vi "Custom Aggregation (Flags).vi"(0 "voltage flags? (F)":bool[](array[boolean]), 1 "reset? (F)":bool, 5 "aggregation settings":T1={"interval"=1, "interval unit"=enum."Runs", "synchronization of intervals"=enum."Not synchronized", "algorithm"=enum."Average"}, 9 "system info in":refnum<class "EP System Info.lvclass">, 11 "error in (no error)":errorcluster, 12 "data timestamp":timestamp) -> (4 "aggregated voltage flags":bool[](array[boolean]), 10 "system info out":refnum<class "EP System Info.lvclass">, 13 "aggregated data valid?":bool, 14 "aggregated data timestamp":timestamp, 15 "error out":errorcluster)   [LabVIEW 2014, in "NI_EP_Power Quality.lvlib"]
doc: "Calculates the aggregated minimum, maximum, and averaged or RMS value of an input signal for a specified aggregation interval, according to Class S in IEC 61000-4-30:2008. There is no overlap between aggregation intervals. This VI automatically restarts accumulation at the beginning of the next time interval after the previous interval expires. You must manually select the polymorphic instance you want to use.\n\nThis VI supports measuring single-line and multiple-line systems except the DBL instance. Use the DBL instance to measure one channel on one line at one time."
uses:
  <vilib>/addons/Electrical Power/PQ/NI_EP_Power Quality.lvlib
  <vilib>/addons/Electrical Power/PQ/Common/Controls/ep_Aggregation Settings.ctl
  <vilib>/addons/Electrical Power/PQ/Common/Classes/System Info/EP System Info.lvclass
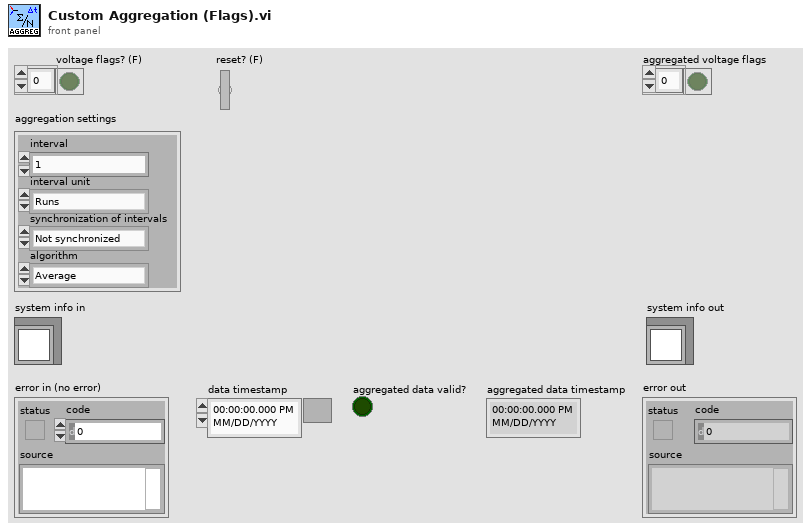
[diagram p1: front panel]
types:
  T1 = typedef "NI_EP_Power Quality.lvlib/ep_Aggregation Settings.ctl" = cluster{"interval":u32, "interval unit":enum16{"Runs", "Seconds", "Minutes", "Hours", "Days", "Weeks"}, "synchronization of intervals":enum16{"Not synchronized", "Interval rounded"}, "algorithm":enum16{"Average", "RMS"}}
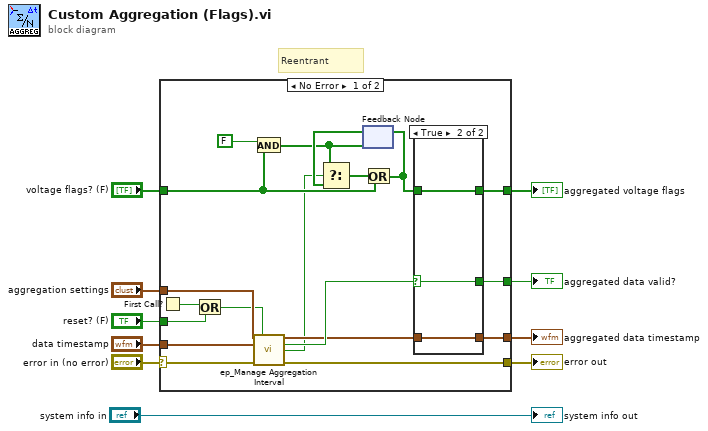
[diagram p0: block diagram]
diagram:
  # "Reentrant"
  n1 = case shown="No Error" "error in (no error)" {
    selector: "error in (no error)" -> [w22 w34]
    tunnel: "voltage flags? (F)" -> [w19 _]
    tunnel: "aggregation settings" -> [w14 _]
    tunnel: "data timestamp" -> [w28 _]
    tunnel: [w27 w34] -> w9
    tunnel: [w21 _] -> w10
    tunnel: [w25 _] -> w2
    tunnel: [w23 _] -> w8
    tunnel: "reset? (F)" -> [w12 _]
    frame No Error {
      n2 = First Call?() -> (First Call?: T/F=w13:bool)
      n3 = Or(x=w13, y=w12) -> (x .or. y?=w11:bool)
      n4 = And(x=FALSE, y=w19) -> (x .and. y?=w20:bool[])
      n5 = call <vilib>:"ep_Manage Aggregation Interval.vi"("aggregation settings"=w14, "restart (F)"=w11, "data time stamp"=w28, "error in (no error)"=w22) -> ("aggregated data time stamp"=w24:timestamp, "aggregated data valid?"=w26:bool, "restart aggregation?"=w15:bool, "error out"=w27:errorcluster)  [unwired: 7 in, 1 out]
      n6 = feedback #1(w20) -> (w29:bool[])
      n7 = Select(t=w20, s=w15, f=w29) -> (s? t:f=w18:bool[])
      n8 = Or(x=w18, y=w19) -> (x .or. y?=w16:bool[])
      n9 = feedback-in #1(w16) -> ()
      n10 = case shown="True" w26 {
        selector: w26 -> [w30 w31]
        tunnel: w16 -> [_ w33]
        tunnel: [_ w33] -> w25
        tunnel: w24 -> [_ w32]
        tunnel: [_ w32] -> w23
        tunnel: [w30 w31] -> w21
        frame False {
        }
        frame True {
        }
      }
    }
    frame Error {
    }
  }
  "aggregated voltage flags" <- w2
  "error out" <- w9
  "aggregated data valid?" <- w10
  "aggregated data timestamp" <- w8
  "system info out" <- "system info in"
